vi "CRYView Pic Get CurverOutList.vi"() -> (0 "bResult":bool, 2 "cCurverOutData_Out":T1)   [LabVIEW 2013]
uses:
  CRYView Global.vi
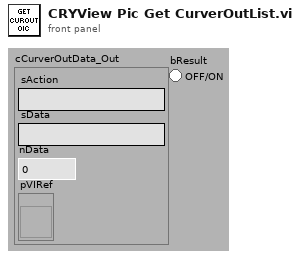
[diagram p1: front panel]
types:
  T1 = cluster{"sAction":string, "sData":string, "nData":i32, "pVIRef":refnum<vi>}
  T2 = cluster{"sAction":string, "sData":string, "nData":i32, "pVIRef":refnum<vi>}[]
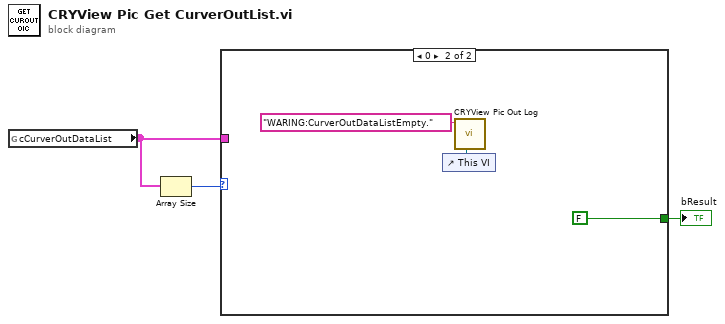
[diagram p0: block diagram]
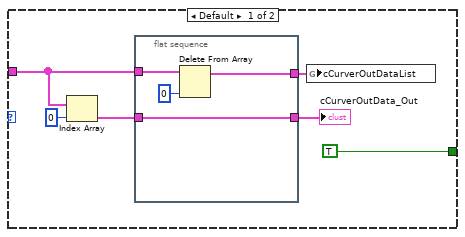
[diagram p2: hidden frame]
diagram:
  n1 = global read "CRYView Global.vi" "cCurverOutDataList"() -> (w2:T2)
  n2 = Array Size(array=w2) -> (size(s)=w3:i32)
  n3 = case shown="0" w3 {
    tunnel: w2 -> [w8 _]
    tunnel: [TRUE FALSE] -> w1
    frame Default {
      n4 = Index Array(array=w8, index=0) -> (element=w7:T1)
      n5 = flat-sequence {
        tunnel: w8 -> [w13]
        tunnel: w7 -> [w10]
        tunnel: [w11] -> w6
        tunnel: [w10] -> w5
        frame #0 {
          n6 = Delete From Array(array=w13, index=0) -> (array with subset deleted=w11:T2)  [unwired: 1 in, 1 out]
        }
      }
      n7 = global write "CRYView Global.vi" "cCurverOutDataList"(w6) -> ()
      "cCurverOutData_Out" <- w5
    }
    frame 0 {
      n8 = control-ref of="This VI"() -> (w15:refnum<vi>)
      n9 = call "CRYView Pic Out Log.vi"("vi reference"=w15, "sData"="WARING:CurverOutDataListEmpty.") -> ()  [unwired: 10 in]
    }
  }
  "bResult" <- w1
